vi "Open Next File.vi"(5 "Input File Pattern":string="Test", 6 "Dir Path":path) -> (0 "Error Message":string, 2 "File Ref Num":refnum<file>, 3 "Output File Name":string, 4 "Stop":bool)   [LabVIEW 2020]
doc: "This VI takes a file name and keeps incrementing a tail until it can open a file that does not already exist. Scott Hannahs, FBNML, Jan 1992"
uses:
  <vilib>/Utility/error.llb/DialogType.ctl
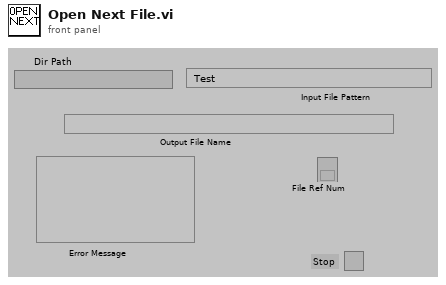
[diagram p1: front panel]
types:
  T1 = typedef "DialogType.ctl" = u16
  T2 = enum16{"open", "replace", "create", "open or create", "replace or create", "replace or create with confirmation"}
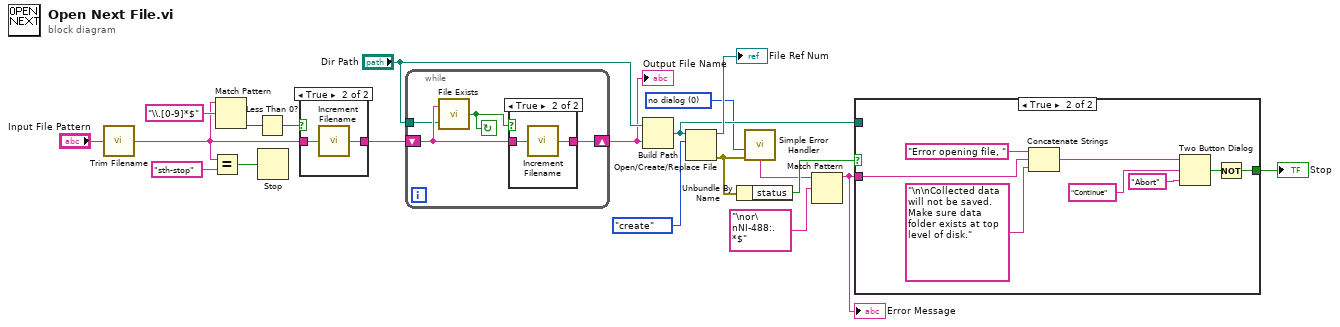
[diagram p0: block diagram]
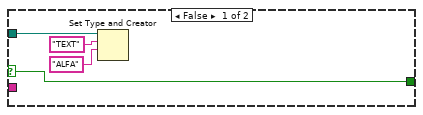
[diagram p3: hidden frame]
diagram:
  w1 = T1 0 items=["no dialog", "OK message", "continue or stop message", "OK message + warnings", "continue/stop + warnings"] ("type of dialog (OK msg:1)")
  n1 = call "Trim Filename.vi"("Input String"="Input File Pattern") -> ("Ouptput String"=w12:string)
  n2 = Equal?(x=w12, y="sth-stop") -> (x = y?=w10:bool)
  n3 = Match Pattern(string=w12, regular expression="\\.[0-9]*$") -> (offset past match=w20:i32)  [unwired: 1 in, 3 out]
  n4 = Less Than 0?(x=w20) -> (x < 0?=w19:bool)
  n5 = Stop(stop? (T)=w10) -> ()
  n6 = case shown="True" w19 {
    tunnel: [w21 w22] -> w17
    tunnel: w12 -> [w21 w23]
    frame False {
    }
    frame True {
      n7 = call "Increment Filename.vi"("Filename In"=w23) -> ("Filename Out"=w22:string)
    }
  }
  n8 = while {
    tunnel: "Dir Path" -> [w24]
    shift-left: w17 -> [w25]
    shift-right: [w26] -> w15
    stop <- w27 continue-if-true
    n9 = call "File Exists.vi"("Dir Path"=w24, "FILESPEC"=w25) -> (0:w27:bool)
    n10 = case shown="True" w27 {
      tunnel: w25 -> [w28 w29]
      tunnel: [w28 w30] -> w26
      frame False {
      }
      frame True {
        n11 = call "Increment Filename.vi"("Filename In"=w29) -> ("Filename Out"=w30:string)
      }
    }
  }
  "Output File Name" <- w15
  n12 = Build Path(base path="Dir Path", name or relative path=w15) -> (appended path=w9:path)
  n13 = Open/Create/Replace File(file path (use dialog)=w9, operation (0:open)=T2."create") -> (refnum out=→"File Ref Num":refnum<file>, error out=w7:errorcluster)  [unwired: 4 in, 1 out]
  n14 = Unbundle By Name(w7) -> ("status"=w6:bool)
  n15 = call <vilib>:"Simple Error Handler.vi"("type of dialog (OK msg:1)"=w1, "error in (no error)"=w7) -> ("message"=w4:string)  [unwired: 3 in, 4 out]
  n16 = Match Pattern(string=w4, regular expression="\nor\nNI-488:.*$") -> (before substring=w3:string)  [unwired: 1 in, 3 out]
  "Error Message" <- w3
  n17 = case shown="True" w6 {
    selector: w6 -> [w31 _]
    tunnel: w9 -> [w34 _]
    tunnel: [w31 w39] -> w8
    tunnel: w3 -> [_ w38]
    frame False {
      n18 = Set Type and Creator(5:"ALFA", 6:"TEXT", 7:w34) -> ()  [unwired: 1 in, 2 out]
    }
    frame True {
      n19 = Concatenate Strings("Error opening file, ", w38, "\n\nCollected data will not be saved.  Make sure data folder exists at top level of disk.") -> (w35:string)
      n20 = Two Button Dialog(message=w35, 1:"Abort", 2:"Continue") -> (T button?=w41:bool)
      n21 = Not(x=w41) -> (.not. x?=w39:bool)
    }
  }
  "Stop" <- w8
